vi "Message Window GUI.vi"() -> ()   [LabVIEW 2022 SP3, in "stillnessHelper.lvclass"]
uses:
  stillnessHelper.lvclass
panel:
  in  "Message":string="\nPlease Wait...\n\nProcessing!"
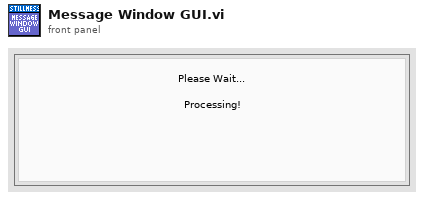
[diagram p1: front panel]
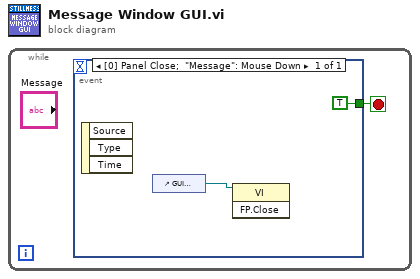
[diagram p0: block diagram]
diagram:
  n1 = while {
    stop <- w1 stop-if-true
    n2 = event shown="[0] Panel Close;  \"Message\": Mouse Down" {
      selector: _ -> [_]
      dyn-events: _ -> [_]
      timeout: _ -> [_]
      tunnel: [TRUE] -> w1
      event Panel Close; "Message": Mouse Down {
        n3 = event-data() -> ()  [unwired: 1 in, 3 out]
        n4 = control-ref of="GUI Reference"() -> (w2:refnum<vi>)
        n5 = invoke class="VI" method="FP.Close"(reference=w2) -> ()  [unwired: 2 in, 3 out]
      }
    }
  }
